vi "Close TCP Connection.vi"(1 "abort (F)":bool, 2 "connection ID":refnum<k5>) -> (0 "error out":errorcluster)   [LabVIEW 2011]
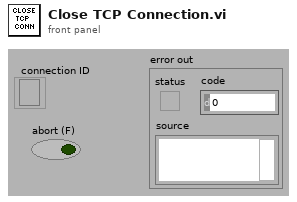
[diagram p1: front panel]
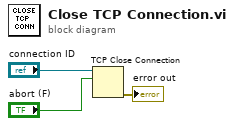
[diagram p0: block diagram]
diagram:
  n1 = TCP Close Connection(connection ID="connection ID", abort (F)="abort (F)") -> (error out=→"error out":errorcluster)  [unwired: 1 in, 1 out]
